vi "Save Transport TDMS File.vi"(8 "error in (no error)":errorcluster, 10 "append?":bool, 11 "Control Experiment":refnum<class "SMO.Control Experiment.lvclass">) -> (0 "error out":errorcluster, 3 "Control Experiment out":refnum<class "SMO.Control Experiment.lvclass">)   [LabVIEW 2019, in "SMO.Control Experiment.lvclass"]
uses:
  SMO.Control Experiment.lvclass
  <userlib>/LevyLab/LV-Data/LV-Data/LV-Data.lvclass
  <userlib>/LevyLab/LV-Data/LV-Data/Typedefs/File Type--enum.ctl
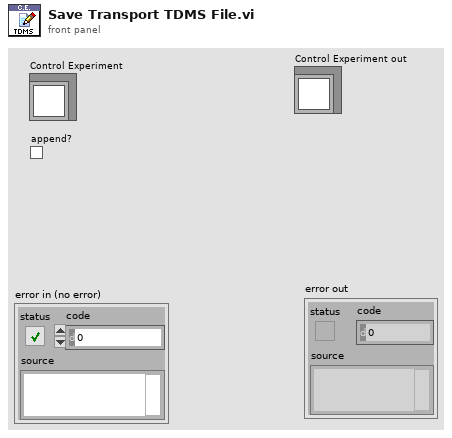
[diagram p1: front panel]
types:
  T1 = typedef "LV-Data.lvclass/File Type--enum.ctl" = enum16{"DAT", "ITX", "TDMS", "VI"}
  T2 = typedef "LV-Data.lvclass/Dictionary--cluster.ctl" = cluster{"key":string, "value":variant}
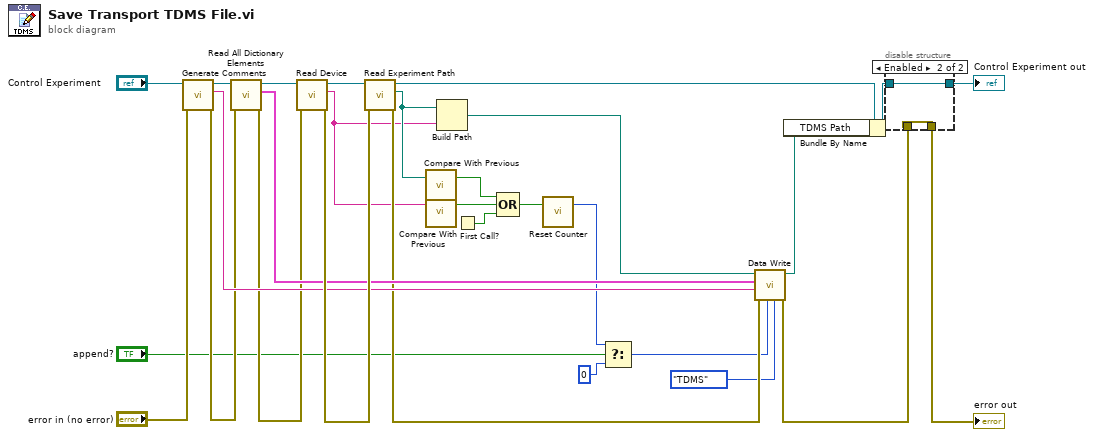
[diagram p0: block diagram]
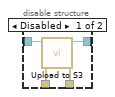
[diagram p2: hidden frame]
diagram:
  n1 = call "Generate Comments.vi"("error in (no error)"="error in (no error)", "Control Experiment"="Control Experiment") -> ("error out"=w22:errorcluster, "Comments"=w26:string, "Control Experiment out"=w25:refnum<class "SMO.Control Experiment.lvclass">)  [unwired: 6 in]
  n2 = call "Read All Dictionary Elements.vi"("error in (no error)"=w22, "Control Experiment"=w25) -> ("error out"=w21:errorcluster, "items"=w27:T2[], "Control Experiment out"=w24:refnum<class "SMO.Control Experiment.lvclass">)  [unwired: 7 in]
  n3 = call "Read Device.vi"("error in (no error)"=w21, "Control Experiment"=w24) -> ("error out"=w28:errorcluster, "Device"=w12:string, "Control Experiment out"=w29:refnum<class "SMO.Control Experiment.lvclass">)  [unwired: 7 in]
  n4 = call "Read Experiment Path.vi"("error in (no error)"=w28, "Control Experiment"=w29) -> ("error out"=w20:errorcluster, "Experiment Path"=w15:path, "Control Experiment out"=w5:refnum<class "SMO.Control Experiment.lvclass">)  [unwired: 7 in]
  n5 = call "Compare With Previous.vi"("Variant"=w15) -> ("Not Equal?"=w10:bool)  [unwired: 2 in]
  n6 = call "Compare With Previous.vi"("Variant"=w12) -> ("Not Equal?"=w11:bool)  [unwired: 2 in]
  n7 = Build Path(base path=w15, name or relative path=w12) -> (appended path=w8:path)
  n8 = First Call?() -> (First Call?: T/F=w14:bool)
  n9 = Compound Arithmetic op=OR(w10, w11, w14) -> (w13:bool)
  n10 = call "Reset Counter.vi"("Reset"=w13) -> ("Counter"=w9:i32)  [unwired: 2 in]
  n11 = Select(t=w9, s="append?", f=0 ("Append Index")) -> (s? t:f=w16:i32)
  n12 = call <userlib>:"Data Write.vi"("File Type"=File_Type--enum."TDMS", "Append Index"=w16, "error in (no error)"=w20, "Notes"=w26, "Data (Dictionary)"=w27, "path"=w8) -> ("error out"=w2:errorcluster, "path out"=w6:path)  [unwired: 4 in]
  n13 = Bundle By Name(cluster=w5, "TDMS Path"=w6) -> (w4:refnum<class "SMO.Control Experiment.lvclass">)
  n14 = disable-structure shown="Enabled" {
    disable-tunnel: w4 -> [w33 w35]
    disable-tunnel: [w32 w35] -> w3
    disable-tunnel: w2 -> [w31 w34]
    disable-tunnel: [w30 w34] -> w1
    frame Disabled {
      n15 = call "Upload to S3.vi"("error in (no error)"=w31, "Control Experiment"=w33) -> ("error out"=w30:errorcluster, "Control Experiment out"=w32:refnum<class "SMO.Control Experiment.lvclass">)  [unwired: 8 in]
    }
    frame Enabled {
    }
  }
  "error out" <- w1
  "Control Experiment out" <- w3
